vi "Convert Position Real to Target.vi"(5 "PPR":dbl=1024.0 format="%#_13g", 7 "Zero Value":dbl, 11 "Real Position":dbl) -> (3 "Position (0-1)":dbl)   [LabVIEW 2023, in "Thor-SwerveDrive_ACT.lvlib"]
uses:
  Thor-SwerveDrive_ACT.lvlib
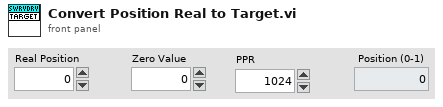
[diagram p1: front panel]
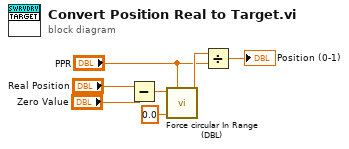
[diagram p0: block diagram]
diagram:
  n1 = Subtract(x="Real Position", y="Zero Value") -> (x-y=w7:dbl)
  n2 = call "Force circular In Range (DBL).vi"("Max"="PPR", "Min"=0.0 ("y"), "Value"=w7) -> ("Value Out"=w6:dbl)  [unwired: 7 in, 1 out]
  n3 = Divide(x=w6, y="PPR") -> (x/y=→"Position (0-1)":dbl)
